vi "AttrSetListenOnly.vi"(5 "LogSuspend":bool, 8 "error in":errorcluster, 10 "Enabled":bool, 11 "UdsHandleIn":T1={"LogPath"=path "", "LogEnabled"=FALSE, "isOpen"=FALSE, "LogContent"="", "Adapter"="CAN0", "MCanHandle"={"MCanAdapter"=refnum}, "TransmittId"=0, "ReceiveId"=0}) -> (0 "error out":errorcluster, 3 "UdsHandleOut":T1={"LogPath"=path "", "LogEnabled"=FALSE, "isOpen"=FALSE, "LogContent"="", "Adapter"="CAN0", "MCanHandle"={"MCanAdapter"=refnum}, "TransmittId"=0, "ReceiveId"=0})   [LabVIEW 2011, in "Konvolucio MUDS150628.lvlib"]
uses:
  <instrlib>/Konvolucio MUDS150628/Konvolucio MUDS150628.lvlib
  <instrlib>/Konvolucio MUDS150628/Types/UdsHandleType.ctl
  <instrlib>/Konvolucio MCAN120803/Types/MCanHandleType.ctl
  C:/Program Files/National Instruments/LabVIEW 2011/instr.lib/Konvolucio MCAN120803/Private/Konvolucio.MCAN120803.dll
  Konvolucio MCAN120803/Private/Konvolucio.MCAN120803.dll
  <instrlib>/Konvolucio MCAN120803/Konvolucio MCAN120803.lvlib
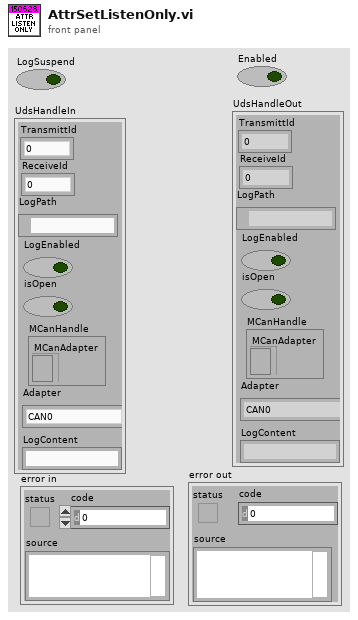
[diagram p1: front panel]
types:
  T1 = typedef "Konvolucio MUDS150628.lvlib/UdsHandleType.ctl" = cluster{"LogPath":path, "LogEnabled":bool, "isOpen":bool, "LogContent":string, "Adapter":string, "MCanHandle":T2, "TransmittId":u32, "ReceiveId":u32}
  T2 = typedef "Konvolucio MCAN120803.lvlib/MCanHandleType.ctl" = cluster{"MCanAdapter":refnum<k24>}
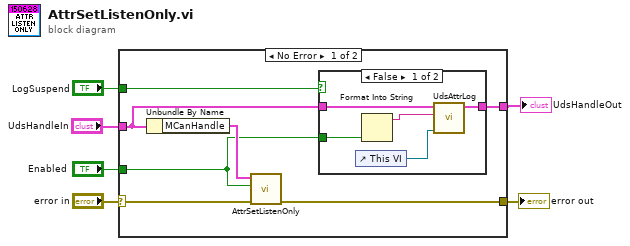
[diagram p0: block diagram]
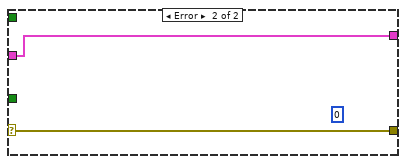
[diagram p3: hidden frame]
diagram:
  n1 = case shown="No Error" "error in" {
    selector: "error in" -> [w9 w21]
    tunnel: [w10 w21] -> w2
    tunnel: "UdsHandleIn" -> [w12 w20]
    tunnel: [w13 w20] -> w5
    tunnel: "LogSuspend" -> [w11 _]
    tunnel: "Enabled" -> [w7 _]
    frame No Error {
      n2 = Unbundle By Name(w12) -> ("MCanHandle"=w8:T2)
      n3 = call <instrlib>:"AttrSetListenOnly.vi"("error in"=w9, "Enabled"=w7, "MCanHandleIn"=w8) -> ("error out"=w10:errorcluster)  [unwired: 6 in, 1 out]
      n4 = case shown="False" w11 {
        tunnel: [w18 w19] -> w13
        tunnel: w12 -> [w16 w19]
        tunnel: w7 -> [w14 _]
        frame False {
          n5 = control-ref of="This VI"() -> (w17:refnum<vi>)
          n6 = Format Into String(w14) -> (resulting string=w15:string)  [unwired: 3 in, 1 out]
          n7 = call <instrlib>:"UdsAttrLog.vi"("This VI"=w17, "Content"=w15, "UdsHandleIn"=w16) -> ("UdsHandleOut"=w18:T1)  [unwired: 8 in]
        }
        frame True {
        }
      }
    }
    frame Error {
      (unwired) u32 0 ("Attributes.RxErrorCounter")
    }
  }
  "error out" <- w2
  "UdsHandleOut" <- w5
